vi "PM5000_Harmonics_Results_Config.vi"(8 "error in":errorcluster, 10 "Seleccion Armonicos":T1(radio), 11 "Network Path":string="172.22.26.202") -> (0 "error out":errorcluster, 3 "Network Path out":string="192.168.169.1")   [LabVIEW 2018]
doc: "Lee la tabla de memoria RealTime_VIF_Power del equipo PowerMonitor 5000, ademas filtra y ordena las variables de interez de la tabla de memoria.\n\nLee las siguientes variables de la tabla RealTime_VIF_Power:\n\n*V1_V2_Volts\n*V2_V3_Volts\n*V3_V1_Volts\n*I1_Amps\n*I2_Amps\n*I3_Amps\n*Frequency_Hz\n*Total_kW\n*Total_kVAR\n*Total_kVA\n*Total_True_PF\n*Total_Disp_PF"
uses:
  <vilib>/RAFA Solutions/Harmony UI Controls Kit/Boolean/Radio Button.ctl
  <vilib>/ethernetip/ethernetip.llb/EthernetIP SLC500 Write Integer.vi
  <vilib>/ethernetip/ethernetip.lvlib
  <vilib>/RAFA Solutions/Harmony UI Controls Kit/Flat UI Design.lvlib
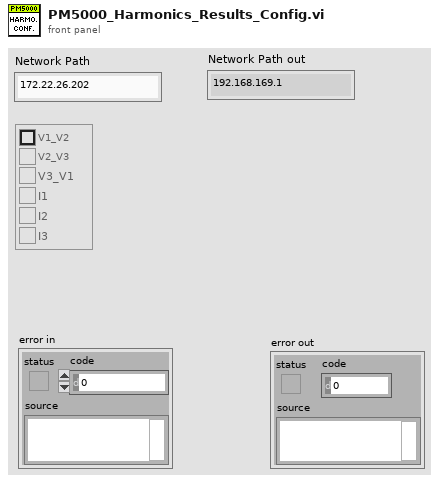
[diagram p1: front panel]
types:
  T1 = enum32{"V1_V2", "V2_V3", "V3_V1", "I1", "I2", "I3"}
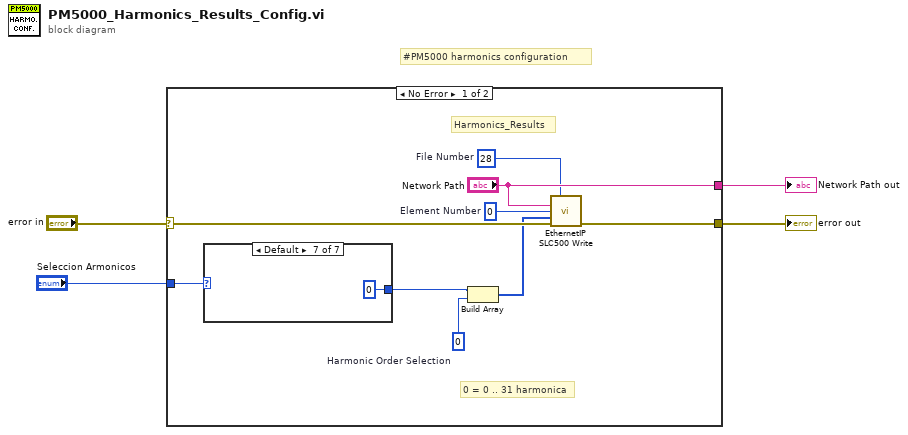
[diagram p0: block diagram]
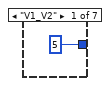
[diagram p2: hidden frame]
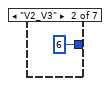
[diagram p3: hidden frame]
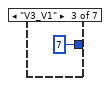
[diagram p4: hidden frame]
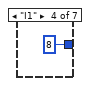
[diagram p5: hidden frame]
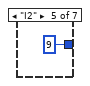
[diagram p6: hidden frame]
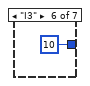
[diagram p7: hidden frame]
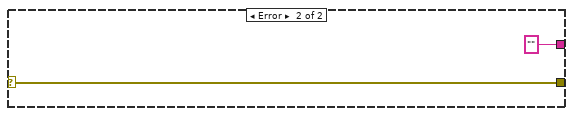
[diagram p8: hidden frame]
diagram:
  # "#PM5000 harmonics configuration"
  n1 = case shown="No Error" "error in" {
    selector: "error in" -> [w11 w22]
    tunnel: [w12 w22] -> w4
    tunnel: ["Network Path" "" ("Network Path")] -> w2
    tunnel: "Seleccion Armonicos" -> [w6 _]
    frame No Error {
      w9 = u16 0  # Harmonic Order Selection
      w7 = u16 28  # File Number
      w13 = u16 0  # Element Number
      # "0 = 0 .. 31 harmonica"
      # "Harmonics_Results"
      n2 = case shown="Default" w6 {
        tunnel: [5 6 7 8 9 10 0] -> w5
        frame "V1_V2" {
        }
        frame "V2_V3" {
        }
        frame "V3_V1" {
        }
        frame "I1" {
        }
        frame "I2" {
        }
        frame "I3" {
        }
        frame Default {
        }
      }
      n3 = Build Array(w5, w9) -> (w8:i32[])
      n4 = call-poly <vilib>:"EthernetIP SLC500 Write.vi"("File Number"=w7, "Network Path"="Network Path", "Element Number"=w13, "Data"=w8, "error in"=w11) -> ("error out"=w12:errorcluster)  [unwired: 9 in, 1 out]
    }
    frame Error {
    }
  }
  "error out" <- w4
  "Network Path out" <- w2
